vi "Demo 1 - Image Gallery - Get Refs to Dynamic VIs.vi"(8 "Error In":errorcluster, 11 "Root Path In":path) -> (0 "Error Out":errorcluster, 3 "Array":refnum<vi>[](array[refnum]))   [LabVIEW 2011]
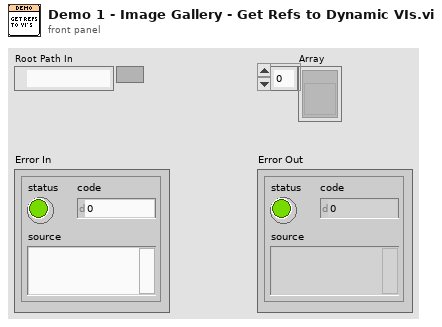
[diagram p1: front panel]
types:
  T1 = enum16{"Always On", "Always Off", "Off While Running"}
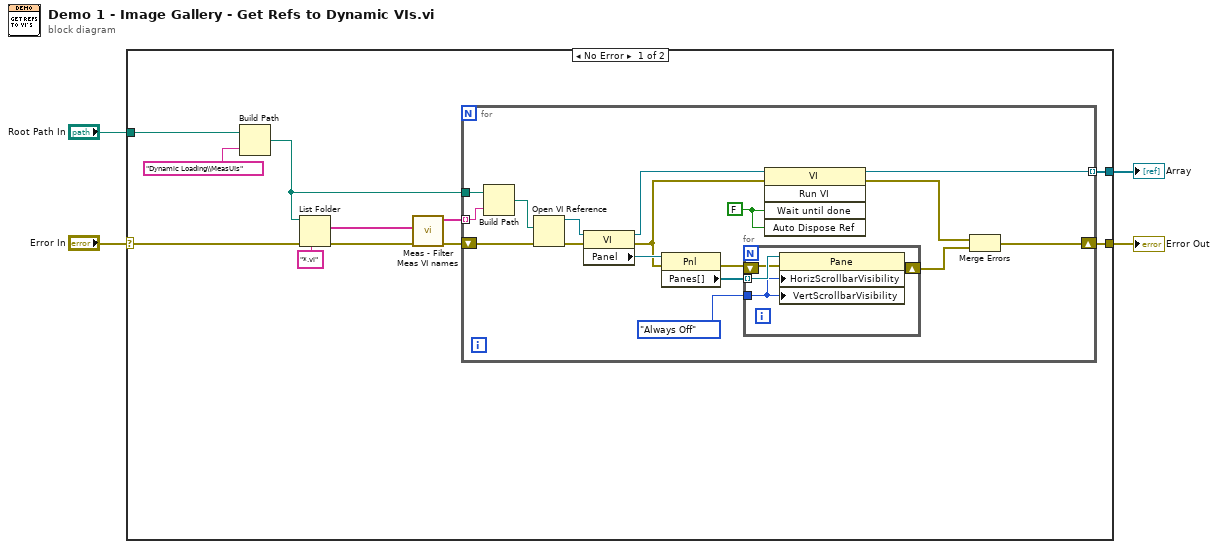
[diagram p0: block diagram]
diagram:
  n1 = case shown="No Error" "Error In" {
    selector: "Error In" -> [w9 w37]
    tunnel: [w15 _] -> w4
    tunnel: "Root Path In" -> [w13 _]
    tunnel: [w10 w37] -> w2
    frame No Error {
      n2 = Build Path(base path=w13, name or relative path="Dynamic Loading\\MeasUIs") -> (appended path=w14:path)
      n3 = List Folder(path=w14, pattern="*.vi", error in=w9) -> (filenames=w6:string[], error out=w7:errorcluster)  [unwired: 1 in, 2 out]
      n4 = call "Meas - Filter Meas VI names.vi"("error in"=w7, "filenames In"=w6) -> ("Error Out"=w5:errorcluster, "Meas VIs Out"=w8:string[])  [unwired: 8 in]
      n5 = for {
        tunnel: w14 -> [w32]
        tunnel: [w23] -> w15 mode=indexing
        shift-right: [w17] -> w10
        shift-left: w5 -> [w27]
        tunnel: w8 -> [w16] mode=indexing
        w22 = FALSE ("Wait Until Done")
        n6 = Build Path(base path=w32, name or relative path=w16) -> (appended path=w28:path)
        n7 = Open VI Reference(vi path=w28, error in (no error)=w27) -> (vi reference=w24:refnum<vi>, error out=w26:errorcluster)  [unwired: 4 in]
        n8 = property class="VI"(reference=w24, error in=w26) -> (reference out=w25:refnum<vi>, error out=w20:errorcluster, "Panel"=w29:refnum<vi>)
        n9 = property class="Pnl"(reference=w29, error in=w20) -> (error out=w21:errorcluster, "Panes[]"=w30:refnum<vi>[])  [unwired: 1 out]
        n10 = for {
          tunnel: w30 -> [w36] mode=indexing
          tunnel: T1."Always Off" ("Horizontal Scrollbar Visibility") -> [w35]
          shift-right: [w33] -> w18
          shift-left: w21 -> [w34]
          n11 = property class="Pane"(reference=w36, error in=w34, "HorizScrollbarVisibility"=w35, "VertScrollbarVisibility"=w35) -> (error out=w33:errorcluster)  [unwired: 1 out]
        }
        n12 = invoke class="VI" method="Run VI"(reference=w25, error in=w20, "Wait until done"=w22, "Auto Dispose Ref"=w22) -> (reference out=w23:refnum<vi>, error out=w19:errorcluster)  [unwired: 1 in, 3 out]
        n13 = Merge Errors(w19, w18) -> (w17:errorcluster)
      }
    }
    frame Error {
    }
  }
  "Array" <- w4
  "Error Out" <- w2
